vi "GPS Processing Module.vi"(0 "FPGA VI Reference In":refnum<k20>, 1 "Arm":enum32{"meArm", "uArm"}(ring), 2 "Servo Motors Control":T1={"Base"=244, "Elbow"=244, "Claw"=244, "Shoulder"=244} {"Shoulder" max=2250 scale=0.0..200.0; "Claw" max=2250 scale=145.0..175.0; "Elbow" max=2250 scale=0.0..200.0; "Base" max=2250 scale=0.0..200.0}, 5 "Coordinates In":T3, 7 "Cluster":cluster{"Time Zone":i32}, 9 "VISA resource name In":refnum<visa-resource-name>, 11 "Error In":errorcluster) -> (3 "Data Valid?":bool, 4 "FPGA VI Reference Out":refnum<k20>, 6 "Error Out":T2, 10 "VISA resource name Out":refnum<visa-resource-name>, 12 "Coordinates Out":T4, 14 "Speed":string, 15 "Error Out":errorcluster)   [LabVIEW 2015]
uses:
  Utilities/Error.ctl
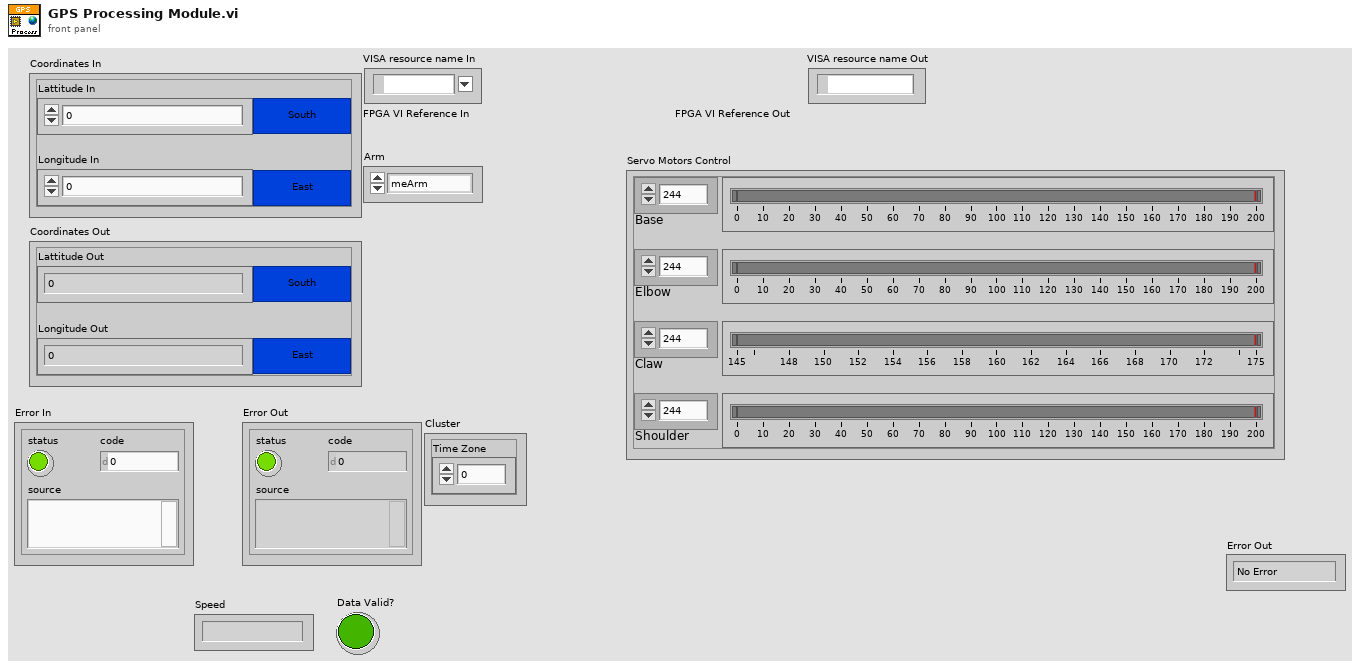
[diagram p1: front panel]
types:
  T1 = cluster{"Base":u16, "Elbow":u16, "Claw":u16, "Shoulder":u16}
  T2 = typedef "Error.ctl" = enum16{"No Error", "Custom", "Standard", "GPS Signal", "YH Left", "YL Right", "XL Back", "XH Front"}
  T3 = cluster{"Lattitude In":dbl, "La I":bool, "Longitude In":dbl, "Lo I":bool}
  T4 = cluster{"Lattitude Out":i32, "La O":bool, "Longitude Out":i32, "Lo O":bool}
  T5 = cluster{"Motor Speed Left":i16, "Motor Speed Right":i16}
  T6 = enum16{"Stop", "LED", "Front", "Back", "Left", "Right"}
  T7 = cluster{"Back":bool, "Front Left":bool, "Front Right":bool}
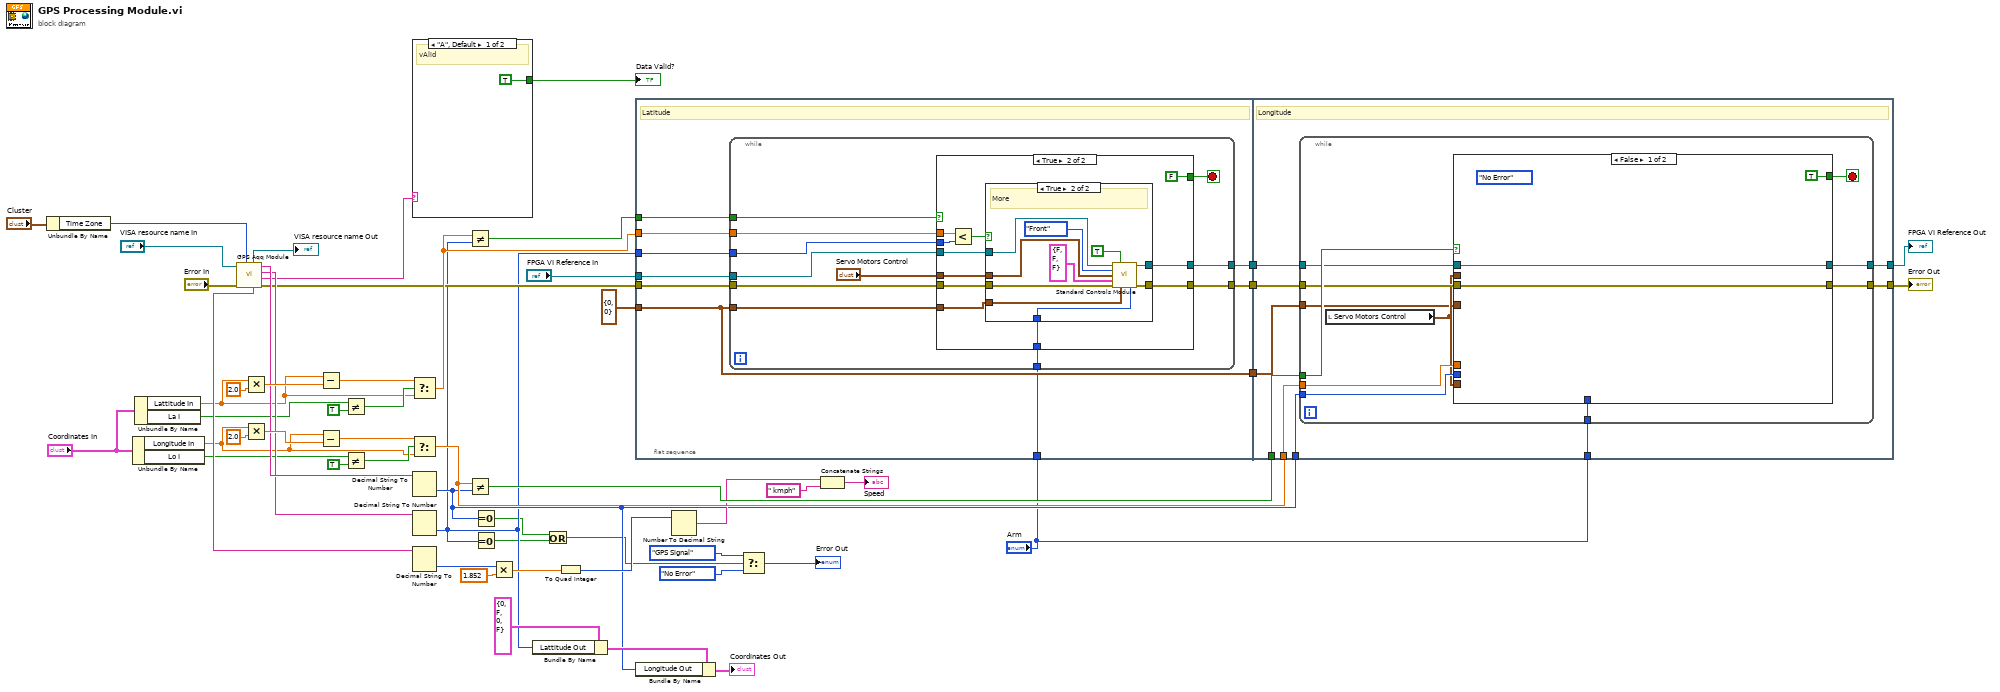
[diagram p0: block diagram]
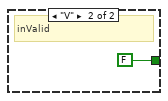
[diagram p2: hidden frame]
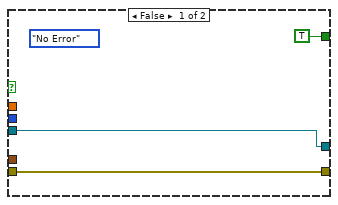
[diagram p3: hidden frame]
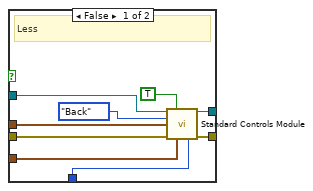
[diagram p4: hidden frame]
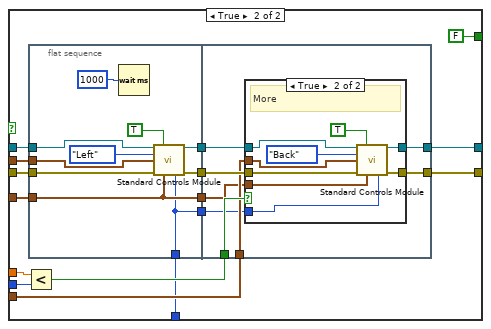
[diagram p5: hidden frame]
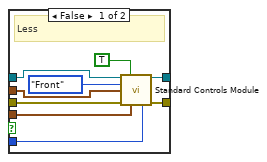
[diagram p6: hidden frame]
diagram:
  n1 = Unbundle By Name("Cluster") -> ("Time Zone"=w19:i32)
  n2 = Unbundle By Name("Coordinates In") -> ("Longitude In"=w25:dbl, "Lo I"=w24:bool)
  n3 = Unbundle By Name("Coordinates In") -> ("Lattitude In"=w27:dbl, "La I"=w26:bool)
  n4 = call "GPS Aqq Module.vi"("time zone"=w19, "Error In"="Error In", "VISA resource name In"="VISA resource name In") -> ("Error Out"=w17:errorcluster, "Status"=w31:string, "Latitude [deg]"=w36:string, "Longitude [deg]"=w37:string, "Speed over ground [knots]"=w40:string, "VISA resource name Out"=→"VISA resource name Out":refnum<visa-resource-name>)  [unwired: 3 in]
  n5 = Multiply(x=w27, y=2.0) -> (x*y=w52:dbl)
  n6 = Multiply(x=w25, y=2.0) -> (x*y=w48:dbl)
  n7 = Subtract(x=w27, y=w52) -> (x-y=w51:dbl)
  n8 = Subtract(x=w25, y=w48) -> (x-y=w47:dbl)
  n9 = Not Equal?(x=w26, y=TRUE) -> (x != y?=w53:bool)
  n10 = Not Equal?(x=w24, y=TRUE) -> (x != y?=w49:bool)
  n11 = case shown="\"A\", Default" w31 {
    tunnel: [TRUE FALSE] -> w30
    frame "A", Default {
      # "vAlid"
    }
    frame "V" {
      # "inValid"
    }
  }
  "Data Valid?" <- w30
  n12 = Select(t=w51, s=w53, f=w27) -> (s? t:f=w44:dbl)
  n13 = Select(t=w47, s=w49, f=w25) -> (s? t:f=w43:dbl)
  n14 = Decimal String To Number(string=w37) -> (number=w15:i32)  [unwired: 2 in, 1 out]
  n15 = Decimal String To Number(string=w36) -> (number=w14:i32)  [unwired: 2 in, 1 out]
  n16 = Decimal String To Number(string=w40) -> (number=w39:i32)  [unwired: 2 in, 1 out]
  n17 = Not Equal?(x=w44, y=w14) -> (x != y?=w56:bool)
  n18 = Not Equal?(x=w43, y=w15) -> (x != y?=w45:bool)
  n19 = Equal To 0?(x=w15) -> (x = 0?=w13:bool)
  n20 = Equal To 0?(x=w14) -> (x = 0?=w12:bool)
  n21 = Multiply(x=w39, y=1.852) -> (x*y=w38:dbl)
  n22 = Bundle By Name(cluster=T4 {"Lattitude Out"=0, "La O"=FALSE, "Longitude Out"=0, "Lo O"=FALSE} ("Coordinates Out"), "Lattitude Out"=w14) -> (w22:T4)
  n23 = Or(x=w13, y=w12) -> (x .or. y?=w11:bool)
  n24 = To Quad Integer(1:w38) -> (0:w35:i64)
  n25 = flat-sequence {
    tunnel: w56 -> [w67]
    tunnel: w44 -> [w66]
    tunnel: w14 -> [w65]
    tunnel: w17 -> [w64]
    tunnel: [w63] -> w29
    tunnel: [w62] -> w16
    tunnel: "FPGA VI Reference In" -> [w61]
    tunnel: T5 {"Motor Speed Left"=0, "Motor Speed Right"=0} ("Speed 2") -> [w60]
    tunnel: [w60] -> w2
    tunnel: "Arm" -> [w59]
    tunnel: w45 -> [w120]
    tunnel: w43 -> [w119]
    tunnel: w15 -> [w118]
    tunnel: [w116] -> w18
    tunnel: w29 -> [w117]
    tunnel: w16 -> [w115]
    tunnel: [w114] -> w5
    tunnel: w2 -> [w113]
    tunnel: "Arm" -> [w112]
    frame #0 {
      # "Latitude"
      n26 = while {
        tunnel: w67 -> [w78]
        tunnel: w66 -> [w76]
        tunnel: w65 -> [w75]
        tunnel: w64 -> [w74]
        tunnel: [w73] -> w63
        tunnel: [w72] -> w62
        tunnel: w61 -> [w70]
        tunnel: w60 -> [w69]
        tunnel: w59 -> [w68]
        stop <- w77 stop-if-true
        n27 = case shown="True" w78 {
          tunnel: [TRUE FALSE] -> w77
          tunnel: w76 -> [_ w90]
          tunnel: w75 -> [_ w89]
          tunnel: w74 -> [w80 w88]
          tunnel: [w80 w87] -> w73
          tunnel: "Servo Motors Control" -> [_ w86]
          tunnel: [w79 w85] -> w72
          tunnel: w70 -> [w79 w84]
          tunnel: w69 -> [_ w83]
          tunnel: w68 -> [_ w82]
          frame False {
            (unwired) enum16{"Standard", "Custom", "No Error"}."No Error" ("Error??")
          }
          frame True {
            n28 = Less?(x=w90, y=w89) -> (x < y?=w91:bool)
            n29 = case shown="True" w91 {
              tunnel: w88 -> [w99 w109]
              tunnel: [w98 w108] -> w87
              tunnel: w86 -> [w97 w107]
              tunnel: [w96 w106] -> w85
              tunnel: w84 -> [w93 w104]
              tunnel: w83 -> [w95 w103]
              tunnel: w82 -> [w94 w102]
              frame False {
                # "Less"
                n30 = call "Standard Controls Module.vi"("FPGA VI Reference In"=w93, "Control Type"=TRUE, "Command"=T6."Back", "Servo Motors Control"=w97, "Error In"=w99, "Speed"=w95, "Arm"=w94) -> ("FPGA VI Reference Out"=w96:refnum<k20>, "Error Out"=w98:errorcluster)  [unwired: 6 in, 1 out]
              }
              frame True {
                # "More"
                n31 = call "Standard Controls Module.vi"("FPGA VI Reference In"=w104, "Control Type"=TRUE, "Command"=T6."Front", "Servo Motors Control"=w107, "Obstacle Data"=T7 {"Back"=FALSE, "Front Left"=FALSE, "Front Right"=FALSE}, "Error In"=w109, "Speed"=w103, "Arm"=w102) -> ("FPGA VI Reference Out"=w106:refnum<k20>, "Error Out"=w108:errorcluster)  [unwired: 5 in, 1 out]
              }
            }
          }
        }
      }
    }
    frame #1 {
      # "Longitude"
      n32 = while {
        tunnel: w120 -> [w131]
        tunnel: w119 -> [w129]
        tunnel: w118 -> [w128]
        tunnel: w117 -> [w127]
        tunnel: [w126] -> w116
        tunnel: w115 -> [w124]
        tunnel: [w123] -> w114
        tunnel: w113 -> [w122]
        tunnel: w112 -> [w121]
        stop <- w130 stop-if-true
        n33 = local read "Servo Motors Control"() -> (w125:T1)
        n34 = case shown="False" w131 {
          tunnel: [TRUE FALSE] -> w130
          tunnel: w129 -> [_ w149]
          tunnel: w128 -> [_ w148]
          tunnel: w127 -> [w133 w147]
          tunnel: [w133 w144] -> w126
          tunnel: w125 -> [_ w143]
          tunnel: w125 -> [_ w142]
          tunnel: w124 -> [w132 w141]
          tunnel: [w132 w139] -> w123
          tunnel: w122 -> [_ w138]
          tunnel: w121 -> [_ w136]
          frame False {
            (unwired) enum16{"Standard", "Custom", "No Error"}."No Error" ("Error??")
          }
          frame True {
            n35 = Less?(x=w149, y=w148) -> (x < y?=w145:bool)
            n36 = flat-sequence {
              tunnel: w147 -> [w156]
              tunnel: [w157] -> w146
              tunnel: w143 -> [w155]
              tunnel: w141 -> [w153]
              tunnel: [w154] -> w140
              tunnel: w138 -> [w152]
              tunnel: [w152] -> w137
              tunnel: w136 -> [w151]
              tunnel: [w151] -> w135
              tunnel: w146 -> [w167]
              tunnel: w145 -> [w168]
              tunnel: [w166] -> w144
              tunnel: w142 -> [w165]
              tunnel: w140 -> [w164]
              tunnel: [w163] -> w139
              tunnel: w137 -> [w162]
              tunnel: w135 -> [w161]
              frame #0 {
                n37 = Wait (ms)(milliseconds to wait=u32 1000) -> ()  [unwired: 1 out]
                n38 = call "Standard Controls Module.vi"("FPGA VI Reference In"=w153, "Control Type"=TRUE, "Command"=T6."Left", "Servo Motors Control"=w155, "Error In"=w156, "Speed"=w152, "Arm"=w151) -> ("FPGA VI Reference Out"=w154:refnum<k20>, "Error Out"=w157:errorcluster)  [unwired: 6 in, 1 out]
              }
              frame #1 {
                n39 = case shown="True" w168 {
                  tunnel: w167 -> [w177 w184]
                  tunnel: [w174 w183] -> w166
                  tunnel: w165 -> [w173 w182]
                  tunnel: w164 -> [w171 w181]
                  tunnel: [w172 w180] -> w163
                  tunnel: w162 -> [w170 w179]
                  tunnel: w161 -> [w169 w178]
                  frame False {
                    # "Less"
                    n40 = call "Standard Controls Module.vi"("FPGA VI Reference In"=w171, "Control Type"=TRUE, "Command"=T6."Front", "Servo Motors Control"=w173, "Error In"=w177, "Speed"=w170, "Arm"=w169) -> ("FPGA VI Reference Out"=w172:refnum<k20>, "Error Out"=w174:errorcluster)  [unwired: 6 in, 1 out]
                  }
                  frame True {
                    # "More"
                    n41 = call "Standard Controls Module.vi"("FPGA VI Reference In"=w181, "Control Type"=TRUE, "Command"=T6."Back", "Servo Motors Control"=w182, "Error In"=w184, "Speed"=w179, "Arm"=w178) -> ("FPGA VI Reference Out"=w180:refnum<k20>, "Error Out"=w183:errorcluster)  [unwired: 6 in, 1 out]
                  }
                }
              }
            }
          }
        }
      }
    }
  }
  n42 = Bundle By Name(cluster=w22, "Longitude Out"=w15) -> (→"Coordinates Out":T4)
  n43 = Number To Decimal String(number=w35) -> (decimal integer string=w33:string)  [unwired: 1 in]
  n44 = Select(t=Error."GPS Signal" ("Error Out 2"), s=w11, f=Error."No Error" ("Error Out 2")) -> (s? t:f=→"Error Out":T2)
  n45 = Concatenate Strings(w33, " kmph" ("string")) -> (→"Speed":string)
  "Error Out" <- w18
  "FPGA VI Reference Out" <- w5
